vi "ETDMS_DebugError.vi"(8 "error in (no error)":errorcluster, 11 "Message":string) -> (0 "error out":errorcluster)   [LabVIEW 2023, in "Embedded TDMS Logger Engine.lvlib"]
uses:
  Embedded TDMS Logger Engine.lvlib
  <vilib>/NI VeriStand/Custom Device Tools/Custom Device Utility Library/Custom Device Utility Library.lvlib
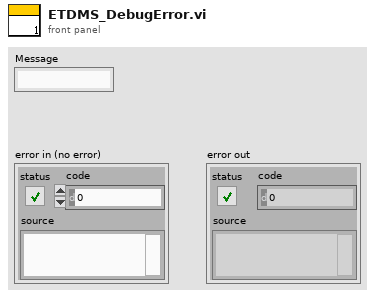
[diagram p1: front panel]
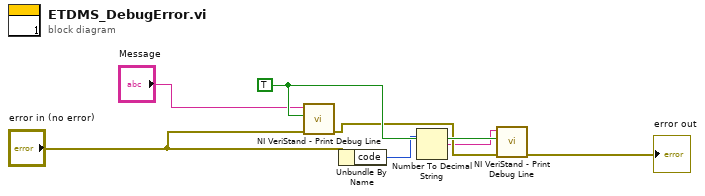
[diagram p0: block diagram]
diagram:
  w6 = TRUE ("Add to log file? (F)")
  n1 = call <vilib>:"NI VeriStand - Print Debug Line.vi"("error in (no error)"="error in (no error)", "Add to log file? (F)"=w6, "Message"="Message") -> ("error out"=w5:errorcluster)  [unwired: 8 in]
  n2 = Unbundle By Name("error in (no error)") -> ("code"=w3:i32)
  n3 = Number To Decimal String(number=w3) -> (decimal integer string=w4:string)  [unwired: 1 in]
  n4 = call <vilib>:"NI VeriStand - Print Debug Line.vi"("error in (no error)"=w5, "Add to log file? (F)"=w6, "Message"=w4) -> ("error out"=→"error out":errorcluster)  [unwired: 8 in]
